vi "ATSh_StartCaptureAsync.vi"(11 "Handle":u32) -> (0 "Return Code":u32)   [LabVIEW 2010]
doc: "_____AlazarTech, Scope_____\n\nStart the Capture of records in the DMA mode."
uses:
  ATSApi.dll
panel:
  out "Handle_Out":u32
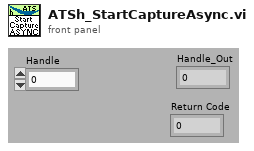
[diagram p1: front panel]
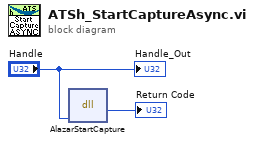
[diagram p0: block diagram]
diagram:
  n1 = dll-call lib="ATSApi.dll" fn="AlazarStartCapture"("Handle"="Handle") -> (→"Return Code":u32)  [unwired: 4 in, 2 out]
  "Handle_Out" <- "Handle"
